vi "GetTrendPointProps.vi"(7 "data event config":T1, 9 "hw status":string, 10 "found hw status":bool, 11 "DataSetName":string) -> (3 "key value pairs out":T4[](array[typedef]))   [LabVIEW 2017, in "EmsaDataEventCreator.lvlib"]
uses:
  <vilib>/addons/InsightCM/Devices/Shared/Emsa/EmsaDataEventCreator/EmsaDataEventCreator.lvlib
  <vilib>/addons/InsightCM/MessageBus/Base/controls/KeyValuePair.ctl
  <vilib>/addons/InsightCM/Devices/Shared/Emsa/EmsaDataEventCreator/controls/DataEventConfig.ctl
  <vilib>/addons/PointValueMap/controls/PointMap.ctl
  <vilib>/addons/InsightCM/Devices/Shared/Emsa/EmsaDataEventCreator/controls/SweepParams.ctl
  <vilib>/addons/InsightCM/Devices/Shared/Common/DataEvent/controls/DataSetType.ctl
  <vilib>/addons/InsightCM/Utilities/PropertyHelpers/PropertyHelpers.lvlib
  <vilib>/addons/InsightCM/Devices/Shared/Common/DataEventCreator/DataEventCreator.lvlib
  <vilib>/addons/InsightCM/Devices/Shared/Common/DataEvent/DataEvent.lvlib
  <vilib>/addons/PointValueMap/PointValueMap.lvlib
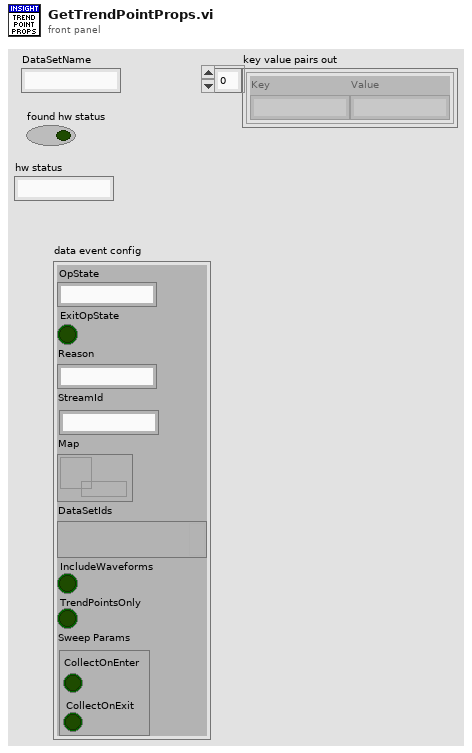
[diagram p1: front panel]
types:
  T1 = typedef "EmsaDataEventCreator.lvlib/DataEventConfig.ctl" = cluster{"OpState":string, "ExitOpState":bool, "Reason":string, "StreamId":string, "Map":T2, "DataSetIds":variant, "IncludeWaveforms":bool, "TrendPointsOnly":bool, "Sweep Params":T3}
  T2 = typedef "PointValueMap.lvlib/PointMap.ctl" = refnum<data-value>
  T3 = typedef "EmsaDataEventCreator.lvlib/SweepParams.ctl" = cluster{"CollectOnEnter":bool, "CollectOnExit":bool}
  T4 = typedef "KeyValuePair.ctl" = cluster{"Key":string, "Value":string}
  T5 = typedef "DataEvent.lvlib/DataSetType.ctl" = enum16{"Waveform", "SpeedProfile", "ThermalImage", "EmsaSweep"}
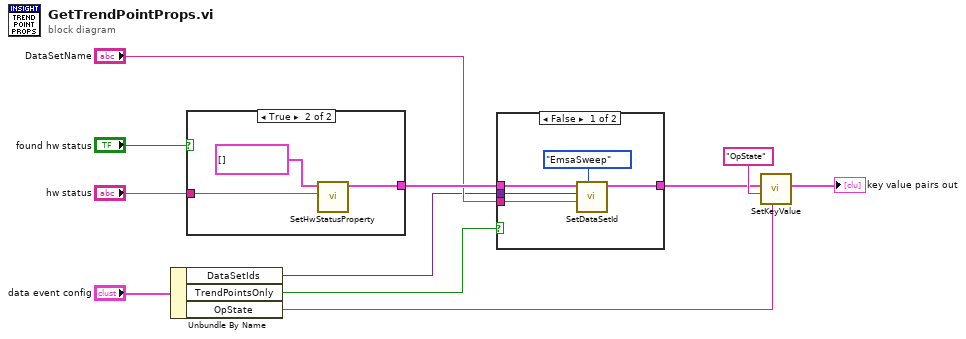
[diagram p0: block diagram]
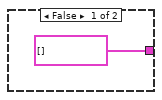
[diagram p3: hidden frame]
diagram:
  n1 = Unbundle By Name("data event config") -> ("DataSetIds"=w1:variant, "TrendPointsOnly"=w2:bool, "OpState"=w4:string)
  n2 = case shown="True" "found hw status" {
    tunnel: [T4[] [] ("props out") w15] -> w10
    tunnel: "hw status" -> [_ w14]
    frame False {
    }
    frame True {
      n3 = call <vilib>:"SetHwStatusProperty.vi"("hw status"=w14, "props in"=T4[] []) -> ("props out"=w15:T4[])  [unwired: 9 in]
    }
  }
  n4 = case shown="False" w2 {
    tunnel: w10 -> [w20 w21]
    tunnel: [w17 w21] -> w7
    tunnel: "DataSetName" -> [w18 _]
    tunnel: w1 -> [w19 _]
    frame False {
      n5 = call <vilib>:"SetDataSetId.vi"("DataSetType"=DataSetType."EmsaSweep", "DataSetName"=w18, "DataSetIds"=w19, "props in"=w20) -> ("props out"=w17:T4[])  [unwired: 7 in]
    }
    frame True {
    }
  }
  n6 = call <vilib>:"SetKeyValue.vi"("value"=w4, "key"="OpState", "key value pairs"=w7) -> ("key value pairs out"=→"key value pairs out":T4[])  [unwired: 8 in]
